vi "getImageCamera.vi"(4 "Mostrar?":bool, 5 "Streeam?":bool, 6 "Image Device IN":cluster{"Image":T1, "errorImage":errorcluster}, 7 "Camera Device IN":T2) -> (1 "Contraste OUT":dbl, 2 "Image Device OUT":cluster{"Image":T1, "errorImage":errorcluster}, 3 "Camara Device OUT":T2)   [LabVIEW 2010]
uses:
  <vilib>/vision/Image Controls.llb/IMAQ Image.ctl
  <vilib>/vision/NI_Vision_Development_Module.lvlib
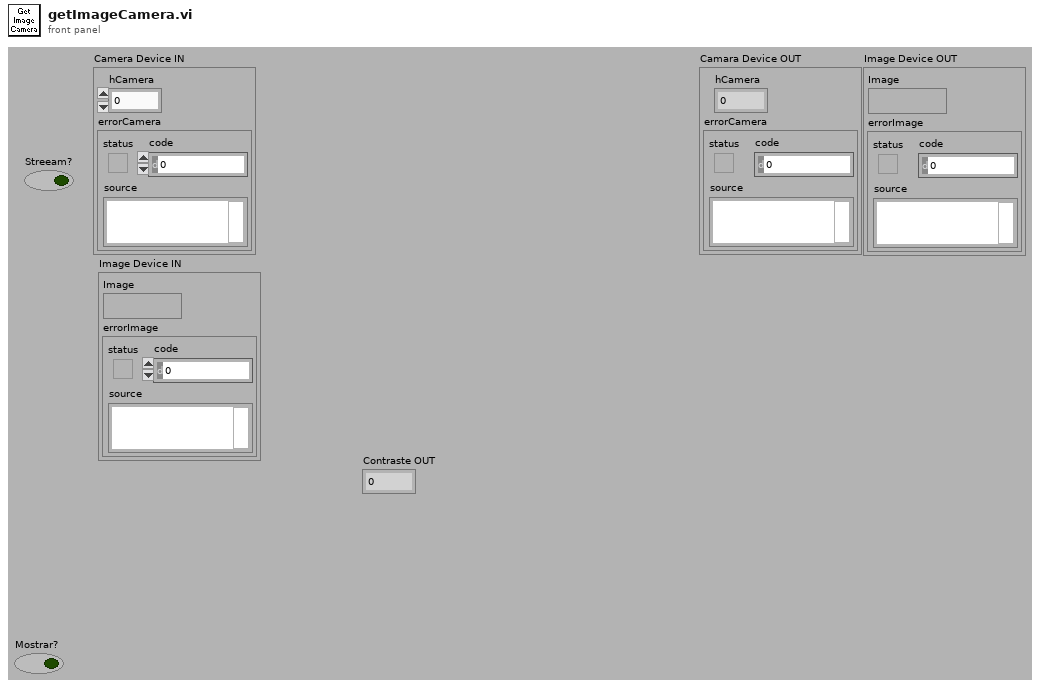
[diagram p1: front panel]
types:
  T1 = typedef "IMAQ Image.ctl" = refnum<image>
  T2 = cluster{"hCamera":u32, "errorCamera":errorcluster}
  T3 = cluster{"Red (or Hue) value":u8, "Green (or Sat) value":u8, "Blue (or Light or Val) value":u8}[]
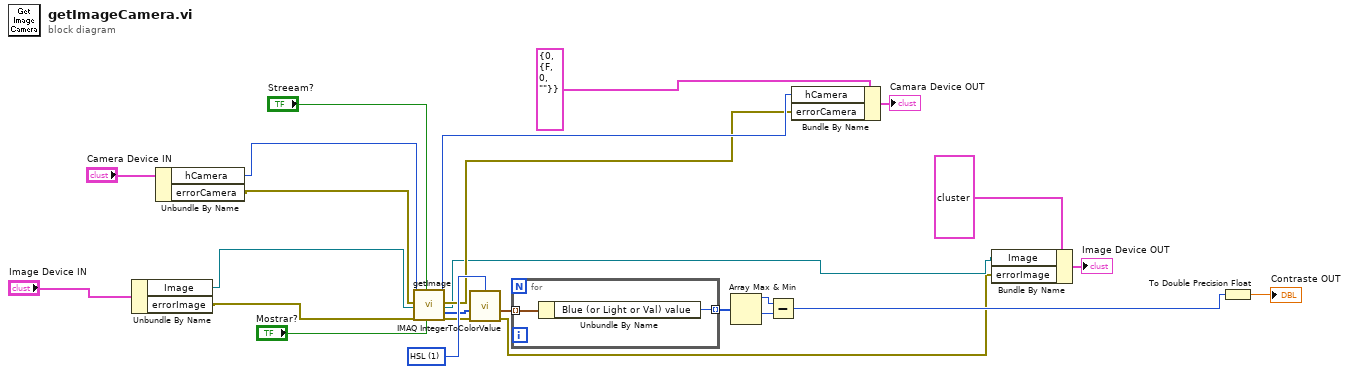
[diagram p0: block diagram]
diagram:
  w21 = u16 1 items=["RGB", "HSL", "HSV", "HSI"] ("Color Mode")
  n1 = Unbundle By Name("Image Device IN") -> ("Image"=w10:T1, "errorImage"=w9:errorcluster)
  n2 = Unbundle By Name("Camera Device IN") -> ("hCamera"=w13:u32, "errorCamera"=w12:errorcluster)
  n3 = call "getImage.vi"("hCamera IN"=w13, "errorCamera IN"=w12, "Image IN"=w10, "imageError IN"=w9, "Streeam"="Streeam?", "Show"="Mostrar?") -> ("hCamera OUT"=w7:u32, "errorCamera OUT"=w6:errorcluster, "Image OUT"=w3:T1, "1D RGB32 Array OUT"=w19:u32[], "errorImage OUT"=w20:errorcluster)  [unwired: 8 in, 1 out]
  n4 = call "IMAQ IntegerToColorValue"("error in (no error)"=w20, "1D U32 array"=w19, "Color Mode"=w21) -> ("1D Color value array"=w22:T3, "error out"=w2:errorcluster)  [unwired: 2 in, 2 out]
  n5 = for {
    tunnel: w22 -> [w27] mode=indexing
    tunnel: [w26] -> w23 mode=indexing
    n6 = Unbundle By Name(w27) -> ("Blue (or Light or Val) value"=w26:u8)
  }
  n7 = Array Max & Min(array=w23) -> (max value=w24:u8, min value=w25:u8)  [unwired: 2 out]
  n8 = Subtract(x=w24, y=w25) -> (x-y=w15:u8)
  n9 = Bundle By Name(cluster=T2 {"hCamera"=0, "errorCamera"={"status"=FALSE, "code"=0, "source"=""}} ("Camera Device"), "hCamera"=w7, "errorCamera"=w6) -> (→"Camara Device OUT":T2)
  n10 = Bundle By Name(cluster=cluster{"Image":T1, "errorImage":errorcluster} {"Image"=refnum, "errorImage"={"status"=FALSE, "code"=0, "source"=""}} ("Image Device"), "Image"=w3, "errorImage"=w2) -> (→"Image Device OUT":cluster{"Image":T1, "errorImage":errorcluster})
  n11 = To Double Precision Float(number=w15) -> (double precision float=→"Contraste OUT":dbl)
